vi "Access insert values.vi"(5 "是否创建唯一键":bool, 6 "Password":string, 7 "data":variant[](array[variant]), 8 "error in (no error)":errorcluster, 9 "columns外部输入":T1, 10 "database":string="database1.mdb", 11 "table":string) -> (0 "error out":errorcluster)   [LabVIEW 2016, in "Access Lib.lvlib"]
uses:
  Access Lib.lvlib
  <vilib>/addons/database/Auxilliary.llb/DB Tools Transaction.ctl
  <vilib>/addons/database/Auxilliary.llb/DB Tools Isolation Level.ctl
  <vilib>/addons/database/Auxilliary.llb/DB Tools Column Info.ctl
  <vilib>/addons/database/Auxilliary.llb/DB Tools DataTypes.ctl
  <vilib>/addons/database/Auxilliary.llb/DB Tools Parameter Info.ctl
  <vilib>/addons/database/Auxilliary.llb/DB Tools Parameter Dir.ctl
  <vilib>/addons/database/Connection.llb/DB Tools Open Connec (String).vi
  <vilib>/addons/database/Connection.llb/Conn Transaction.vi
  <vilib>/addons/database/Connection.llb/Conn Execute.vi
  <vilib>/addons/database/Recordset.llb/Rec Destroy - Connection.vi
  <vilib>/addons/database/Command.llb/Cmd Set Parameter Value (C).vi
  <vilib>/addons/database/Command.llb/Cmd Execute.vi
  <vilib>/addons/database/Recordset.llb/Rec Destroy - Command.vi
  <vilib>/addons/database/Command.llb/Cmd Delete.vi
  <vilib>/addons/database/NI_Database_API.lvlib
  <vilib>/Utility/VariantDataType/VariantType.lvlib
panel:
  out "当前数据时间":timestamp
  out "当前测量模式":string
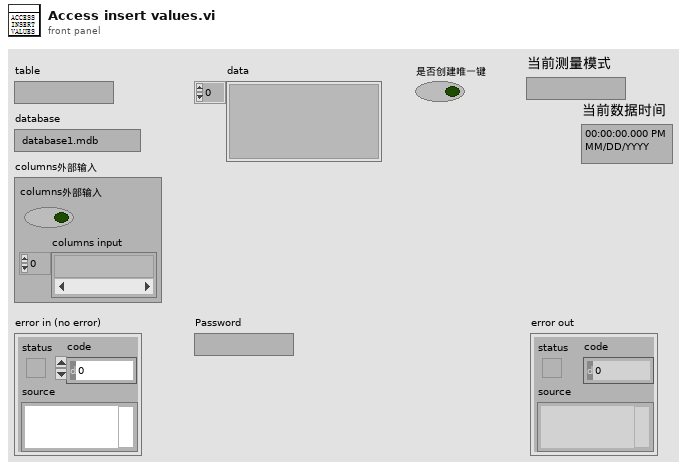
[diagram p1: front panel]
types:
  T1 = cluster{"columns外部输入":bool, "columns input":string[]}
  T2 = typedef "NI_Database_API.lvlib/DB Tools Isolation Level.ctl" = enum16{"chaos", "read uncommitted", "read committed", "repeatable read", "serializable"}
  T3 = typedef "NI_Database_API.lvlib/DB Tools Transaction.ctl" = enum16{"begin", "commit", "rollback"}
  T4 = typedef "NI_Database_API.lvlib/DB Tools Column Info.ctl" = cluster{"column name":string, "data type":T5, "size":i32, "allow null?":bool}
  T5 = typedef "NI_Database_API.lvlib/DB Tools DataTypes.ctl" = enum16{"String", "Long (I32)", "Single (SGL)", "Double (DBL)", "Date/Time", "Binary"}
  T6 = typedef "VariantType.lvlib/Type.ctl" = enum8{"Invalid Type", "Void", "I8", "I16", "I32", "I64", "U8", "U16", "U32", "U64", "Single Float", "Double Float", "Extended Float", "Single Complex", "Double Complex", "Extended Complex", "Enum U8", "Enum U16", "Enum U32", "Enum U64", "Single Float With Unit", "Double Float With Unit", "Extended Float With Unit", "Single Complex with Unit", "Double Complex with Unit", "Extended Complex with Unit", "Boolean", "String", "Path", "Picture", "Tag", "Array", "Cluster", "Variant", "LV Variant", "Waveform", "Timestamp", "Digital Waveform", "Digital Data", "ExpressData", "Refnum", "External Data", "VI", "Poly VI", "LabVIEW Class Instance", "Fixed Point"}
  T7 = typedef "NI_Database_API.lvlib/Conn ObjectReference.ctl" = refnum<k1>
  T8 = typedef "NI_Database_API.lvlib/DB Tools Parameter Info.ctl" = cluster{"parameter name":string, "type":T5, "direction":T9, "value":variant}
  T9 = typedef "NI_Database_API.lvlib/DB Tools Parameter Dir.ctl" = enum32{"Input", "Output", "Input/Output", "Return Value"}
  T10 = typedef "NI_Database_API.lvlib/Rec ObjectReference.ctl" = refnum<k1>
  T11 = typedef "LVDateTimeRec.ctl" = cluster{"秒数的小数部分":dbl, "秒":i32, "分":i32, "时":i32, "日":i32, "月":i32, "年":i32, "天数（周）":i32, "天数（年）":i32, "DST":i32}
  T12 = typedef "NI_Database_API.lvlib/Cmd ObjectReference.ctl" = refnum<k1>
  T13 = typedef "NI_Database_API.lvlib/Cmd-Rec Object Reference.ctl" = refnum<k1>
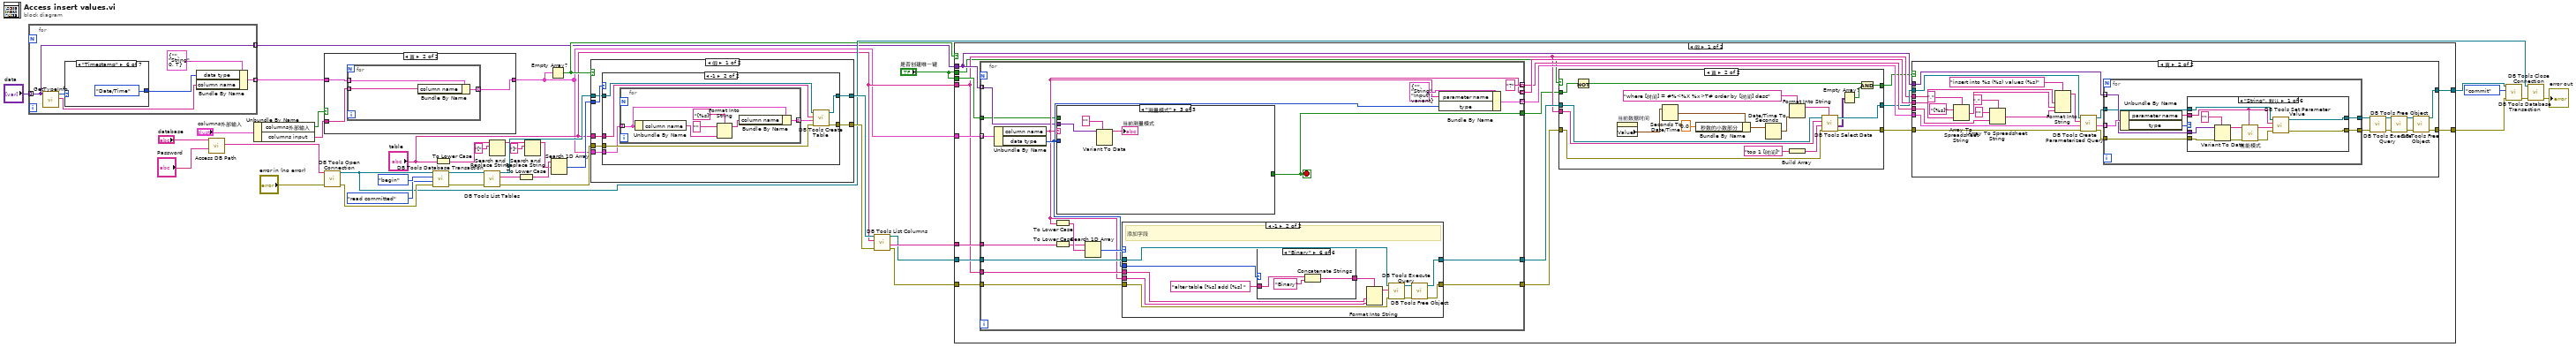
[diagram p0: block diagram]
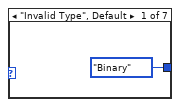
[diagram p3: hidden frame]
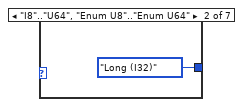
[diagram p4: hidden frame]
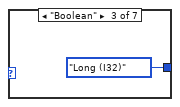
[diagram p5: hidden frame]
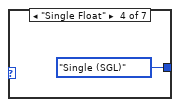
[diagram p6: hidden frame]
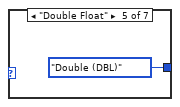
[diagram p7: hidden frame]
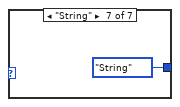
[diagram p8: hidden frame]
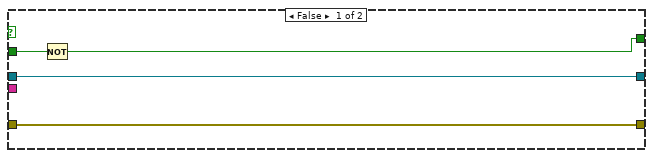
[diagram p11: hidden frame]
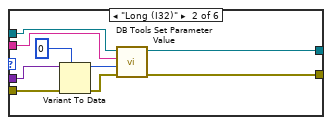
[diagram p13: hidden frame]
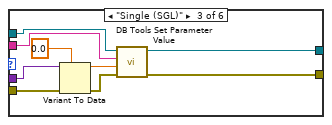
[diagram p14: hidden frame]
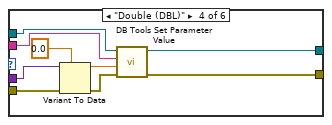
[diagram p15: hidden frame]
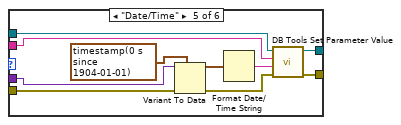
[diagram p16: hidden frame]
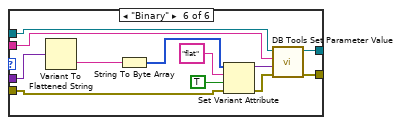
[diagram p17: hidden frame]
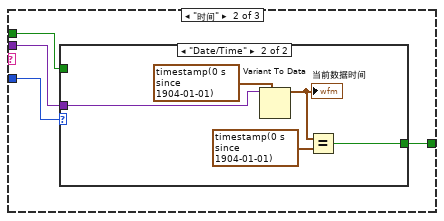
[diagram p19: hidden frame]
diagram:
  n1 = for {
    tunnel: [w41] -> w18 mode=indexing
    tunnel: [w43] -> w15 mode=indexing
    tunnel: "data" -> [w41] mode=indexing
    n2 = call <vilib>:"GetTypeInfo.vi"("Variant"=w41) -> ("Name"=w42:string, "Type Enum"=w45:T6)  [unwired: 6 in, 3 out]
    n3 = case shown="\"Timestamp\"" w45 {
      tunnel: [DB_Tools_DataTypes."Binary" ("data type") DB_Tools_DataTypes."Long (I32)" ("data type") DB_Tools_DataTypes."Long (I32)" ("data type") DB_Tools_DataTypes."Single (SGL)" ("data type") DB_Tools_DataTypes."Double (DBL)" ("data type") DB_Tools_DataTypes."Date/Time" ("data type") DB_Tools_DataTypes."String" ("data type")] -> w44
      frame "Invalid Type", Default {
      }
      frame "I8".."U64", "Enum U8".."Enum U64" {
      }
      frame "Boolean" {
      }
      frame "Single Float" {
      }
      frame "Double Float" {
      }
      frame "Timestamp" {
      }
      frame "String" {
      }
    }
    n4 = Bundle By Name(cluster=T4 {"column name"="", "data type"=enum."String", "size"=0, "allow null?"=TRUE} ("column information"), "data type"=w44, "column name"=w42) -> (w43:T4)
  }
  n5 = call "Access DB Path.vi"("Password"="Password", "database"="database") -> ("Connection information"=w11:string)  [unwired: 8 in, 1 out]
  n6 = Unbundle By Name("columns外部输入") -> ("columns外部输入"=w13:bool, "columns input"=w14:string[])
  n7 = case shown="真" w13 {
    tunnel: w15 -> [w54 w57]
    tunnel: [w54 w56] -> w12
    tunnel: w14 -> [_ w55]
    frame False {
    }
    frame True {
      n8 = for {
        tunnel: w57 -> [w60] mode=indexing
        tunnel: [w59] -> w56 mode=indexing
        tunnel: w55 -> [w58] mode=indexing
        n9 = Bundle By Name(cluster=w60, "column name"=w58) -> (w59:T4)
      }
    }
  }
  n10 = call-poly <vilib>:"DB Tools Open Connection.vi"("error in (no error)"="error in (no error)", "connection information"=w11) -> ("error out"=w25:errorcluster, "connection reference"=w22:T7)  [unwired: 6 in]
  n11 = call-poly <vilib>:"DB Tools Database Transaction.vi"("error in (no error)"=w25, "isolation level (chaos)"=DB_Tools_Isolation_Level."read committed", "operation (begin)"=DB_Tools_Transaction."begin", "connection reference"=w22) -> ("error out"=w24:errorcluster, "connection reference out"=w26:T7)  [unwired: 2 in]
  n12 = To Lower Case(string="table") -> (all lower case string=w6:string)
  n13 = call <vilib>:"DB Tools List Tables.vi"("error in (no error)"=w24, "connection reference"=w26) -> ("error out"=w33:errorcluster, "tables"=w35:string[], "connection reference out"=w23:T7)  [unwired: 3 in]
  n14 = Search and Replace String(input string=w6, search string="[" ("搜索字符串")) -> (result string=w2:string)  [unwired: 6 in, 3 out]
  n15 = To Lower Case(string=w35) -> (all lower case string=w5:string[])
  n16 = Search and Replace String(input string=w2, search string="]" ("搜索字符串")) -> (result string=w3:string)  [unwired: 6 in, 3 out]
  n17 = Empty Array?(array=w12) -> (empty?=w20:bool)
  n18 = Search 1D Array(1D array=w5, element=w3) -> (index of element=w34:i32)  [unwired: 1 in]
  n19 = case shown="假" w20 {
    tunnel: w34 -> [w67 _]
    tunnel: w33 -> [w66 w83]
    tunnel: [w65 w84] -> w31
    tunnel: [w64 w83] -> w30
    tunnel: w23 -> [w63 w84]
    tunnel: "table" -> [w62 _]
    tunnel: w12 -> [w61 _]
    frame False {
      n20 = case shown="-1" w67 {
        tunnel: w63 -> [w69 w76]
        tunnel: w66 -> [w68 w75]
        tunnel: w62 -> [_ w74]
        tunnel: w61 -> [_ w71]
        tunnel: [w69 w73] -> w65
        tunnel: [w68 w72] -> w64
        frame 0, Default {
        }
        frame -1 {
          n21 = for {
            tunnel: w71 -> [w78] mode=indexing
            tunnel: [w77] -> w70 mode=indexing
            n22 = Unbundle By Name(w78) -> ("column name"=w82:string)
            n23 = Format Into String(format string="[%s]" ("格式字符串"), initial string="" ("初始字符串"), w82) -> (resulting string=w79:string)  [unwired: 1 in, 1 out]
            n24 = Bundle By Name(cluster=w78, "column name"=w79) -> (w77:T4)
          }
          n25 = call <vilib>:"DB Tools Create Table.vi"("error in (no error)"=w75, "column information"=w70, "table"=w74, "connection reference"=w76) -> ("error out"=w72:errorcluster, "connection reference out"=w73:T7)  [unwired: 4 in]
        }
      }
    }
    frame True {
    }
  }
  n26 = call <vilib>:"DB Tools List Columns.vi"("error in (no error)"=w30, "table"="table", "connection reference"=w31) -> ("error out"=w9:errorcluster, "columns"=w32:string[], "connection reference out"=w10:T7)  [unwired: 1 in, 1 out]
  n27 = case shown="假" w20 {
    tunnel: w32 -> [w103 _]
    tunnel: w9 -> [w102 w284]
    tunnel: [w98 w285] -> w28
    tunnel: [w97 w284] -> w27
    tunnel: w18 -> [w94 _]
    tunnel: w10 -> [w96 w285]
    tunnel: "table" -> [w88 _]
    tunnel: w12 -> [w95 _]
    tunnel: "是否创建唯一键" -> [w93 _]
    tunnel: "是否创建唯一键" -> [w86 _]
    frame False {
      n28 = for {
        tunnel: w96 -> [w237]
        tunnel: w103 -> [w239]
        tunnel: w102 -> [w236]
        tunnel: [w235] -> w90
        tunnel: w88 -> [w234]
        tunnel: w95 -> [w233] mode=indexing
        tunnel: [w231] -> w101 mode=indexing
        tunnel: [w227] -> w100 mode=indexing
        tunnel: ["?"] -> w99 mode=indexing
        tunnel: [w229] -> w92
        tunnel: w94 -> [w226] mode=indexing
        tunnel: [w225] -> w87
        tunnel: w93 -> [w224]
        stop <- w225 stop-if-true
        n29 = Unbundle By Name(w233) -> ("column name"=w227:string, "data type"=w228:T5)
        n30 = To Lower Case(string=w227) -> (all lower case string=w223:string)
        n31 = To Lower Case(string=w239) -> (all lower case string=w222:string[])
        n32 = case shown="\"测量模式\"" w227 {
          tunnel: w228 -> [_ w243 _]
          tunnel: w226 -> [_ w242 w251]
          tunnel: [_ w241 _] -> w225
          tunnel: w224 -> [_ w240 _]
          frame "假", Default {
          }
          frame "时间" {
            n33 = case shown="\"Date/Time\"" w243 {
              tunnel: w242 -> [_ w248]
              tunnel: [_ w244] -> w241
              tunnel: w240 -> [_ _]
              frame "String", Default {
              }
              frame "Date/Time" {
                n34 = Variant To Data(type=timestamp(0 s since 1904-01-01) ("时间标识"), Variant=w248) -> (data=w246:timestamp)  [unwired: 1 in, 1 out]
                "当前数据时间" <- w246
                n35 = Equal?(x=w246, y=timestamp(0 s since 1904-01-01) ("时间标识")) -> (x = y?=w244:bool)
              }
            }
          }
          frame "测量模式" {
            n36 = Variant To Data(type="", Variant=w251) -> (data=→"当前测量模式":string)  [unwired: 1 in, 1 out]
          }
        }
        n37 = Search 1D Array(1D array=w222, element=w223) -> (index of element=w238:i32)  [unwired: 1 in]
        n38 = case shown="-1" w238 {
          tunnel: [w253 w262] -> w235
          tunnel: w237 -> [w252 w261]
          tunnel: w227 -> [_ w260]
          tunnel: w236 -> [w253 w259]
          tunnel: w234 -> [_ w258]
          tunnel: w228 -> [_ w256]
          tunnel: [w252 w254] -> w229
          frame 0, Default {
          }
          frame -1 {
            # "添加字段"
            n39 = case shown="\"Binary\"" w256 {
              tunnel: "alter table [%s] add [%s] " -> [w268 w271 w274 w277 w280 w283]
              tunnel: [w267 w270 w273 w276 w279 w282] -> w255
              frame "String", Default {
                n40 = Concatenate Strings(w268, "String" ("字符串")) -> (w267:string)
              }
              frame "Long (I32)" {
                n41 = Concatenate Strings(w271, "Long" ("字符串")) -> (w270:string)
              }
              frame "Single (SGL)" {
                n42 = Concatenate Strings(w274, "Single" ("字符串")) -> (w273:string)
              }
              frame "Double (DBL)" {
                n43 = Concatenate Strings(w277, "Double" ("字符串")) -> (w276:string)
              }
              frame "Date/Time" {
                n44 = Concatenate Strings(w280, "TimeStamp" ("字符串")) -> (w279:string)
              }
              frame "Binary" {
                n45 = Concatenate Strings(w283, "Binary" ("字符串")) -> (w282:string)
              }
            }
            n46 = Format Into String(format string=w255, w258, w260) -> (resulting string=w263:string)  [unwired: 2 in, 1 out]
            n47 = call-poly <vilib>:"DB Tools Execute Query.vi"("error in (no error)"=w259, "SQL query"=w263, "connection reference"=w261) -> ("error out"=w264:errorcluster, "recordset reference"=w265:T10)  [unwired: 5 in]
            n48 = call-poly <vilib>:"DB Tools Free Object.vi"("error in (no error)"=w264, "recordset reference"=w265) -> ("error out"=w262:errorcluster, "connection reference"=w254:T7)  [unwired: 8 in]
          }
        }
        n49 = Bundle By Name(cluster=T8 {"parameter name"="", "type"=enum."String", "direction"=enum."Input", "value"=variant} ("parameter information"), "parameter name"=w227, "type"=w228) -> (w231:T8)
      }
      n50 = case shown="真" w86 {
        tunnel: w92 -> [w107 w124]
        tunnel: [w107 w123] -> w91
        tunnel: w90 -> [w106 w122]
        tunnel: [w106 w121] -> w89
        tunnel: w88 -> [_ w120]
        tunnel: w87 -> [w105 w109]
        tunnel: [w104 w111] -> w85
        frame False {
          n51 = Not(x=w105) -> (.not. x?=w104:bool)
        }
        frame True {
          n52 = Not(x=w109) -> (.not. x?=w108:bool)
          n53 = property on="当前数据时间" class="AbsTime (严格)"() -> ("Value"=w117:timestamp)  [unwired: 2 in, 2 out]
          n54 = Seconds To Date/Time(time stamp (now)=w117) -> (date time rec=w116:T11)  [unwired: 1 in]
          n55 = Bundle By Name(cluster=w116, "秒数的小数部分"=0.0) -> (w113:T11)
          n56 = Date/Time To Seconds(2:w113) -> (0:w114:timestamp)  [unwired: 1 in]
          n57 = Format Into String(format string="where [时间] = #%<%X %x>T# order by [时间] desc" ("condition"), w114) -> (resulting string=w119:string)  [unwired: 2 in, 1 out]
          n58 = Build Array("top 1 [时间]") -> (w126:string[])
          n59 = call <vilib>:"DB Tools Select Data.vi"("condition"=w119, "error in (no error)"=w122, "columns"=w126, "table"=w120, "connection reference"=w124) -> ("error out"=w121:errorcluster, "data"=w112:variant[][], "connection reference out"=w123:T7)  [unwired: 1 in]
          n60 = Empty Array?(array=w112) -> (empty?=w110:bool)
          n61 = And(x=w108, y=w110) -> (x .and. y?=w111:bool)
        }
      }
      n62 = case shown="真" w85 {
        tunnel: w101 -> [_ w154]
        tunnel: w100 -> [_ w148]
        tunnel: w99 -> [_ w146]
        tunnel: [w128 w136] -> w98
        tunnel: [w127 w135] -> w97
        tunnel: w91 -> [w128 w133]
        tunnel: w89 -> [w127 w131]
        tunnel: w88 -> [_ w130]
        tunnel: w94 -> [_ w129]
        frame False {
        }
        frame True {
          n63 = Array To Spreadsheet String(delimiter (Tab)="," ("分隔符(Tab)"), array=w148, 3:"[%s]" ("格式字符串")) -> (spreadsheet string=w147:string)
          n64 = Array To Spreadsheet String(delimiter (Tab)="," ("分隔符(Tab)"), array=w146, 3:"" ("格式字符串")) -> (spreadsheet string=w145:string)
          n65 = Format Into String(format string="insert into %s (%s) values (%s)" ("格式字符串"), w130, w147, w145) -> (resulting string=w144:string)  [unwired: 2 in, 1 out]
          n66 = call <vilib>:"DB Tools Create Parameterized Query.vi"("error in (no error)"=w131, "parameters"=w154, "SQL query"=w144, "connection reference"=w133) -> ("error out"=w143:errorcluster, "parameters out"=w142:T8[], "command reference"=w134:T12)  [unwired: 3 in]
          n67 = for {
            tunnel: w134 -> [w159]
            tunnel: w143 -> [w157]
            tunnel: w142 -> [w162] mode=indexing
            tunnel: w129 -> [w160] mode=indexing
            tunnel: [w156] -> w132
            tunnel: [w155] -> w141
            n68 = Unbundle By Name(w162) -> ("parameter name"=w158:string, "type"=w161:T5)
            n69 = case shown="\"String\", 默认" w161 {
              tunnel: w160 -> [w169 w175 w182 w192 w209 w213]
              tunnel: w159 -> [w170 w179 w186 w196 w207 w221]
              tunnel: w158 -> [w163 w178 w185 w191 w202 w220]
              tunnel: w157 -> [w166 w173 w183 w193 w205 w212]
              tunnel: [w168 w177 w187 w195 w204 w219] -> w156
              tunnel: [w167 w176 w184 w194 w203 w218] -> w155
              frame "String", Default {
                n70 = Variant To Data(error in=w166, type="", Variant=w169) -> (data=w165:string, error out=w172:errorcluster)
                n71 = call "性能模式.vi"("colomn"=w163, "数据标识输入"=w165) -> ("数据标识输出"=w164:string)  [unwired: 9 in]
                n72 = call-poly <vilib>:"DB Tools Set Parameter Value.vi"("error in (no error)"=w172, "value"=w164, "parameter index"=w163, "command reference"=w170) -> ("error out"=w167:errorcluster, "command reference out"=w168:T12)  [unwired: 4 in]
              }
              frame "Long (I32)" {
                n73 = Variant To Data(error in=w173, type=0, Variant=w175) -> (data=w180:i32, error out=w181:errorcluster)
                n74 = call-poly <vilib>:"DB Tools Set Parameter Value.vi"("error in (no error)"=w181, "value"=w180, "parameter index"=w178, "command reference"=w179) -> ("error out"=w176:errorcluster, "command reference out"=w177:T12)  [unwired: 4 in]
              }
              frame "Single (SGL)" {
                n75 = Variant To Data(error in=w183, type=sgl 0.0, Variant=w182) -> (data=w189:sgl, error out=w190:errorcluster)
                n76 = call-poly <vilib>:"DB Tools Set Parameter Value.vi"("error in (no error)"=w190, "value"=w189, "parameter index"=w185, "command reference"=w186) -> ("error out"=w184:errorcluster, "command reference out"=w187:T12)  [unwired: 4 in]
              }
              frame "Double (DBL)" {
                n77 = Variant To Data(error in=w193, type=0.0, Variant=w192) -> (data=w198:dbl, error out=w199:errorcluster)
                n78 = call-poly <vilib>:"DB Tools Set Parameter Value.vi"("error in (no error)"=w199, "value"=w198, "parameter index"=w191, "command reference"=w196) -> ("error out"=w194:errorcluster, "command reference out"=w195:T12)  [unwired: 4 in]
              }
              frame "Date/Time" {
                n79 = Variant To Data(error in=w205, type=timestamp(0 s since 1904-01-01) ("时间标识"), Variant=w209) -> (data=w201:timestamp, error out=w206:errorcluster)
                n80 = Format Date/Time String(seconds (now)=w201) -> (date/time string=w200:string)  [unwired: 2 in]
                n81 = call-poly <vilib>:"DB Tools Set Parameter Value.vi"("error in (no error)"=w206, "value"=w200, "parameter index"=w202, "command reference"=w207) -> ("error out"=w203:errorcluster, "command reference out"=w204:T12)  [unwired: 4 in]
              }
              frame "Binary" {
                n82 = Variant To Flattened String(Variant=w213) -> (data string=w214:string)  [unwired: 1 out]
                n83 = String To Byte Array(string=w214) -> (unsigned byte array=w217:u8[])
                n84 = Set Variant Attribute(Variant=w217, name="flat", value=TRUE, error in=w212) -> (Variant out=w210:variant, error out=w211:errorcluster)  [unwired: 1 out]
                n85 = call-poly <vilib>:"DB Tools Set Parameter Value.vi"("error in (no error)"=w211, "value"=w210, "parameter index"=w220, "command reference"=w221) -> ("error out"=w218:errorcluster, "command reference out"=w219:T12)  [unwired: 4 in]
              }
            }
          }
          n86 = call-poly <vilib>:"DB Tools Execute Query.vi"("error in (no error)"=w141, "command reference"=w132) -> ("error out"=w139:errorcluster, "command-recordset reference"=w140:T13)  [unwired: 6 in]
          n87 = call-poly <vilib>:"DB Tools Free Object.vi"("error in (no error)"=w139, "command-recordset reference"=w140) -> ("error out"=w137:errorcluster, "command reference"=w138:T12)  [unwired: 8 in]
          n88 = call-poly <vilib>:"DB Tools Free Object.vi"("error in (no error)"=w137, "command reference"=w138) -> ("error out"=w135:errorcluster, "connection reference"=w136:T7)  [unwired: 8 in]
        }
      }
    }
    frame True {
    }
  }
  n89 = call-poly <vilib>:"DB Tools Database Transaction.vi"("error in (no error)"=w27, "operation (begin)"=DB_Tools_Transaction."commit", "connection reference"=w28) -> ("error out"=w29:errorcluster)  [unwired: 3 in, 1 out]
  n90 = call <vilib>:"DB Tools Close Connection.vi"("error in (no error)"=w29, "connection reference"=w22) -> ("error out"=→"error out":errorcluster)  [unwired: 5 in]
